vi "auto-concatenating-tunnel.vi"() -> ()   [LabVIEW 2025]
panel:
  out "Array 2":i32[](array[numeric])
  out "Array":i32[](array[numeric])
  out "Numeric":i32
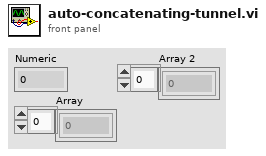
[diagram p1: front panel]
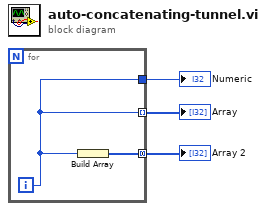
[diagram p0: block diagram]
diagram:
  n1 = for {
    tunnel: [w5] -> w3
    tunnel: [w5] -> w2 mode=indexing
    tunnel: [w4] -> w1 mode=concatenating
    i -> [w5]
    n2 = Build Array(w5) -> (w4:i32[])
  }
  "Numeric" <- w3
  "Array" <- w2
  "Array 2" <- w1
